vi "SECoP_dataCreateInteger.vi"(6 "value":i64, 8 "error in (no error)":errorcluster, 9 "maximum value":i64=9223372036854775807, 10 "minimum value":i64=-9223372036854775807, 11 "DLL path (in)":T2) -> (0 "error out":errorcluster, 2 "SECoP_dataPtr (out)":T1 {"ptr64" format="%.0x"; "ptr32" format="%.0x"}, 3 "DLL path (out)":T2)   [LabVIEW 2023, in "SECoP.lvlib"]
doc: "Call <b>\"SECoP_dataCreateInteger.vi\"</b> to create a simple inetegr (numeric) data type and set value. Free resources after use with <b>\"SECoP_dataDestroy.vi\"</b>.\n\n<b>DLL path</b> input and output of cluster from \"SECoP-Initialize.vi\"\n<b>minimum value</b> smallest allowed value\n<b>maximum value</b> greatest allowed value\n<b>value</b> new value\n<b>SECoP_dataPtr</b> created data"
uses:
  SECoP.lvlib
  SECoP-libraries.ctl
  SECoP-data.ctl
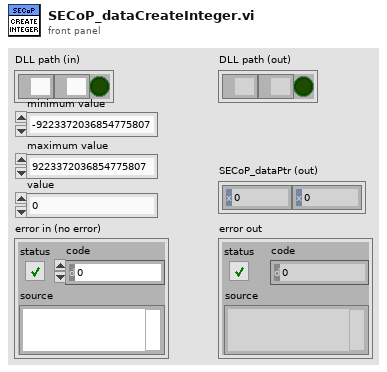
[diagram p1: front panel]
types:
  T1 = typedef "SECoP.lvlib/SECoP-data.ctl" = cluster{"ptr32":u32, "ptr64":u64}
  T2 = typedef "SECoP.lvlib/SECoP-libraries.ctl" = cluster{"serverDLL":path, "variantDLL":path, "cleanup_mode":bool}
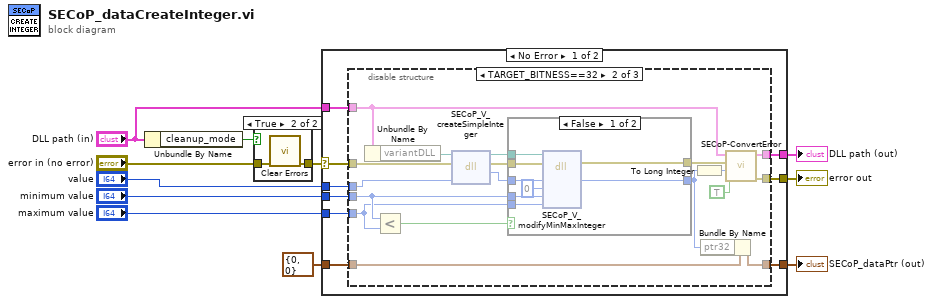
[diagram p0: block diagram]
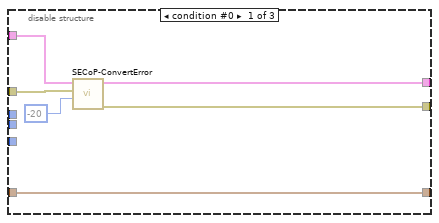
[diagram p3: hidden frame]
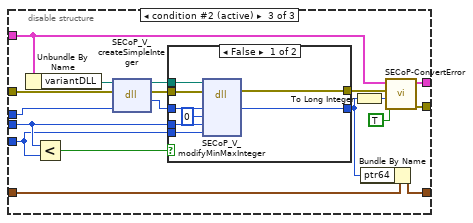
[diagram p5: hidden frame]
diagram:
  n1 = Unbundle By Name("DLL path (in)") -> ("cleanup_mode"=w9:bool)
  n2 = case shown="True" w9 {
    tunnel: "error in (no error)" -> [w12 w14]
    tunnel: [w12 w13] -> w7
    frame False {
    }
    frame True {
      n3 = call <vilib>:"Clear Errors.vi"("error in (no error)"=w14) -> ("error out"=w13:errorcluster)  [unwired: 5 in, 1 out]
    }
  }
  n4 = case shown="No Error" w7 {
    selector: w7 -> [w23 w87]
    tunnel: "DLL path (in)" -> [w22 w88]
    tunnel: [w20 w88] -> w11
    tunnel: [w21 w87] -> w10
    tunnel: [w18 w86] -> w6
    tunnel: T1 {"ptr32"=0, "ptr64"=0} ("SECoP_dataPtr (out)") -> [w19 w86]
    tunnel: "minimum value" -> [w17 _]
    tunnel: "maximum value" -> [w16 _]
    tunnel: "value" -> [w15 _]
    frame No Error {
      n5 = disable-structure shown="TARGET_BITNESS==32" {
        disable-tunnel: w23 -> [w29 w47 w75]
        disable-tunnel: w22 -> [w28 w30 w58]
        disable-tunnel: [w26 w44 w72] -> w21
        disable-tunnel: [w27 w43 w71] -> w20
        disable-tunnel: w19 -> [w24 w45 w73]
        disable-tunnel: [w24 w46 w74] -> w18
        disable-tunnel: w17 -> [_ w35 w63]
        disable-tunnel: w16 -> [_ w34 w62]
        disable-tunnel: w15 -> [_ w32 w60]
        frame condition #0 {
          n6 = call "SECoP-ConvertError.vi"("return code"=-20, "error in (no error)"=w29, "DLL path (in)"=w28) -> ("error out"=w26:errorcluster, "DLL path (out)"=w27:T2)  [unwired: 7 in]
        }
        frame condition #1 {
          n7 = Unbundle By Name(w30) -> ("variantDLL"=w31:path)
          n8 = Less?(x=w35, y=w34) -> (x < y?=w33:bool)
          n9 = dll-call lib="Z:/Praktische_Aufgaben/SECoP-LabVIEW2015/32bit/SECoP32.dll" fn="SECoP_V_createSimpleInteger"(path in=w31, error in=w47, "llValue"=w32) -> (path out=w40:path, error out=w39:errorcluster, "return type"=w37:u32)  [unwired: 2 in]
          n10 = case shown="False" w33 {
            tunnel: w40 -> [w55 _]
            tunnel: w39 -> [w54 w57]
            tunnel: [w53 w57] -> w38
            tunnel: w37 -> [w52 w56]
            tunnel: [w51 w56] -> w36
            tunnel: w35 -> [w49 _]
            tunnel: w34 -> [w48 _]
            frame False {
              n11 = dll-call lib="Z:/Praktische_Aufgaben/SECoP-LabVIEW2015/32bit/SECoP32.dll" fn="SECoP_V_modifyMinMaxInteger"(path in=w55, error in=w54, "pData"=w52, "uPosition"=u32 0, "llMinimum"=w49, "llMaximum"=w48) -> (error out=w53:errorcluster, "pData"=w51:u32)  [unwired: 5 in, 1 out]
            }
            frame True {
            }
          }
          n12 = To Long Integer(number=w36) -> (32bit integer=w41:i32)
          n13 = Bundle By Name(cluster=w45, "ptr32"=w36) -> (w46:T1)
          n14 = call "SECoP-ConvertError.vi"("return is boolean"=TRUE, "return code"=w41, "error in (no error)"=w38, "DLL path (in)"=w30) -> ("error out"=w44:errorcluster, "DLL path (out)"=w43:T2)  [unwired: 6 in]
        }
        frame condition #2 (active) {
          n15 = Unbundle By Name(w58) -> ("variantDLL"=w59:path)
          n16 = Less?(x=w63, y=w62) -> (x < y?=w61:bool)
          n17 = dll-call lib="Z:/Praktische_Aufgaben/SECoP-LabVIEW2015/32bit/SECoP32.dll" fn="SECoP_V_createSimpleInteger"(path in=w59, error in=w75, "llValue"=w60) -> (path out=w68:path, error out=w67:errorcluster, "return type"=w65:u64)  [unwired: 2 in]
          n18 = case shown="False" w61 {
            tunnel: w68 -> [w83 _]
            tunnel: w67 -> [w82 w85]
            tunnel: [w81 w85] -> w66
            tunnel: w65 -> [w80 w84]
            tunnel: [w79 w84] -> w64
            tunnel: w63 -> [w77 _]
            tunnel: w62 -> [w76 _]
            frame False {
              n19 = dll-call lib="Z:/Praktische_Aufgaben/SECoP-LabVIEW2015/32bit/SECoP32.dll" fn="SECoP_V_modifyMinMaxInteger"(path in=w83, error in=w82, "pData"=w80, "uPosition"=u32 0, "llMinimum"=w77, "llMaximum"=w76) -> (error out=w81:errorcluster, "pData"=w79:u64)  [unwired: 5 in, 1 out]
            }
            frame True {
            }
          }
          n20 = To Long Integer(number=w64) -> (32bit integer=w69:i32)
          n21 = Bundle By Name(cluster=w73, "ptr64"=w64) -> (w74:T1)
          n22 = call "SECoP-ConvertError.vi"("return is boolean"=TRUE, "return code"=w69, "error in (no error)"=w66, "DLL path (in)"=w58) -> ("error out"=w72:errorcluster, "DLL path (out)"=w71:T2)  [unwired: 6 in]
        }
      }
    }
    frame Error {
    }
  }
  "DLL path (out)" <- w11
  "error out" <- w10
  "SECoP_dataPtr (out)" <- w6
